vi "Check.vi"(8 "error in (no error)":errorcluster, 10 "Encoded string":string, 11 "Encoding in":refnum<class "CConfig Automatic Encoding.lvclass">) -> (0 "error out":errorcluster, 1 "Match?":bool=TRUE, 2 "Encoded string":string, 3 "Encoding out":refnum<class "CConfig Automatic Encoding.lvclass">)   [LabVIEW 2013, in "CConfig Automatic Encoding.lvclass"]
doc: "Copyright 2018, Carya Automatisering, Wiebe Walstra."
uses:
  CConfig Automatic Encoding.lvclass
  CConfig Automatic Encoding.lvclass/CConfig Automatic Encoding.ctl
  CConfig Encoding.lvclass
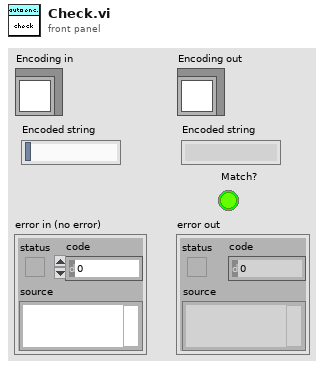
[diagram p1: front panel]
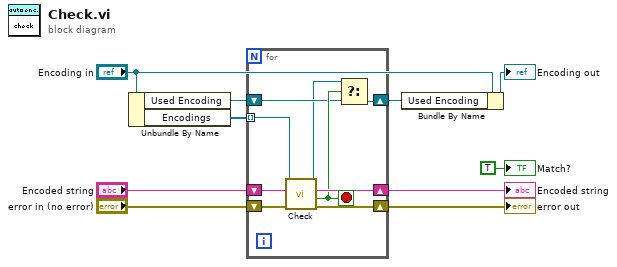
[diagram p0: block diagram]
diagram:
  n1 = Unbundle By Name("Encoding in") -> ("Used Encoding"=w8:refnum<class "CConfig Encoding.lvclass">, "Encodings"=w9:refnum<class "CConfig Encoding.lvclass">[])
  n2 = for {
    tunnel: w9 -> [w17] mode=indexing
    shift-right: [w12] -> w1
    shift-left: w8 -> [w13]
    shift-right: [w18] -> w6
    shift-left: "error in (no error)" -> [w19]
    shift-right: [w15] -> w4
    shift-left: "Encoded string" -> [w16]
    stop <- w14 stop-if-true
    n3 = call-dynamic "Check.vi"("error in (no error)"=w19, "Encoded string"=w16, "Encoding in"=w17) -> ("error out"=w18:errorcluster, "Match?"=w14:bool, "Encoded string"=w15:string, "Encoding out"=w11:refnum<class "CConfig Encoding.lvclass">)  [unwired: 5 in]
    n4 = Select(t=w11, s=w14, f=w13) -> (s? t:f=w12:refnum<class "CConfig Encoding.lvclass">)
  }
  "error out" <- w6
  "Encoded string" <- w4
  n5 = Bundle By Name(cluster="Encoding in", "Used Encoding"=w1) -> (→"Encoding out":refnum<class "CConfig Automatic Encoding.lvclass">)
  "Match?" <- TRUE ("Match?")
